vi "get 2d list.vi"(8 "error in (no error)":errorcluster, 10 "Y":u32[](array[numeric]), 11 "X":u32[](array[numeric])) -> (0 "error out (no error)":errorcluster, 1 "upper limit":dbl[](array[numeric]), 2 "lower limit":dbl[](array[numeric]), 4 "X Values":u32[](array[numeric]))   [LabVIEW 2016]
doc: "Takes X and Y create ROI values and confirms that all x values have two y values"
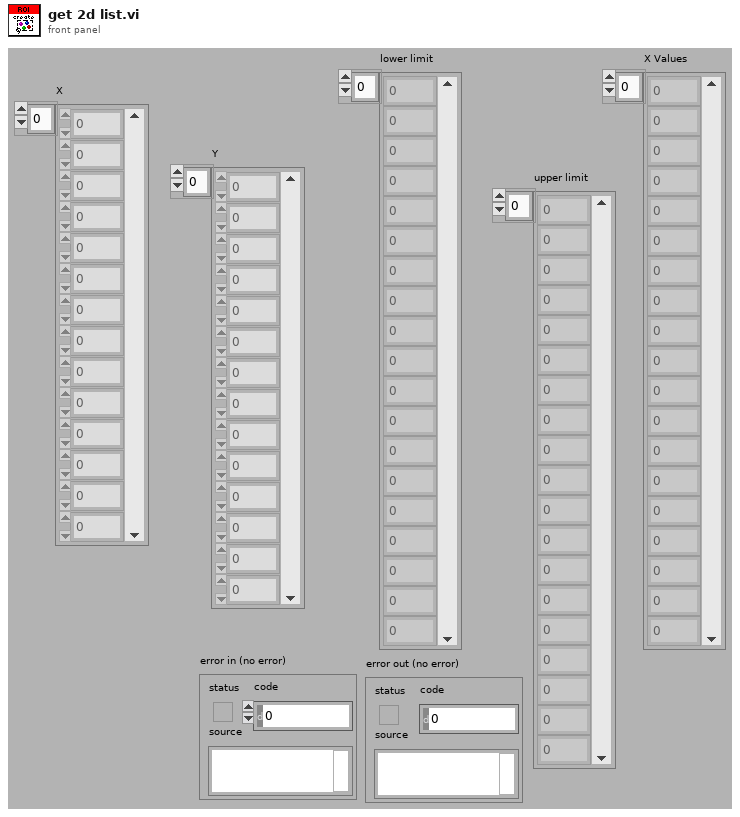
[diagram p1: front panel]
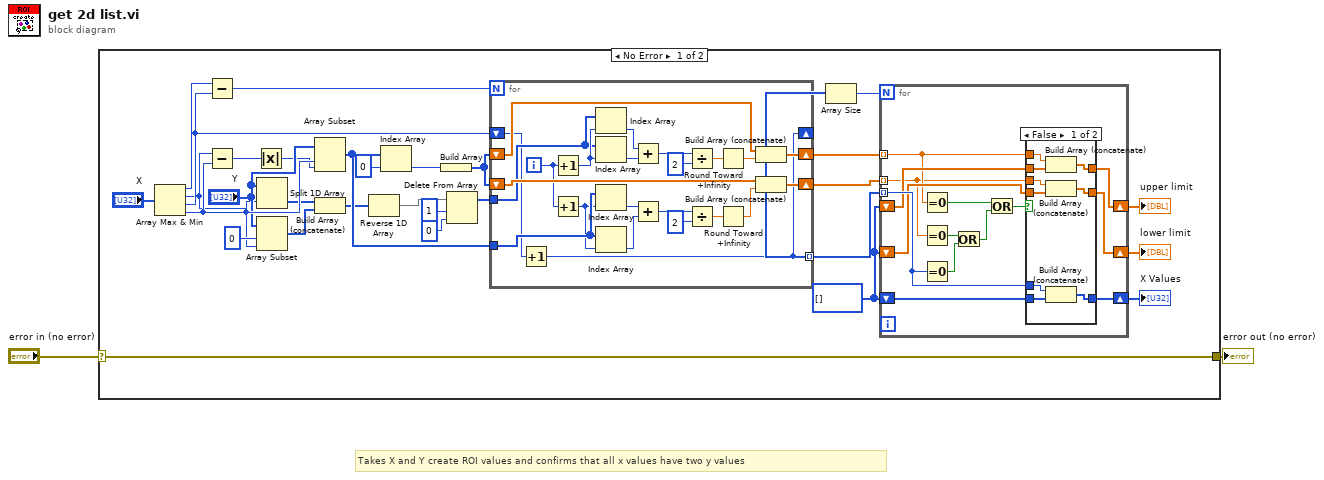
[diagram p0: block diagram]
diagram:
  # "Takes X and Y create ROI values and confirms that all x values have two y values"
  n1 = case shown="No Error" "error in (no error)" {
    selector: "error in (no error)" -> [w3 w82]
    tunnel: [w3 w82] -> w1
    frame No Error {
      w12 = u32[] []
      n2 = Array Max & Min(array="X") -> (max value=w14:u32, max index (indices)=w4:i32, min value=w15:u32, min index (indices)=w27:i32)
      n3 = Subtract(x=w14, y=w15) -> (x-y=w13:u32)
      n4 = Subtract(x=w4, y=w27) -> (x-y=w17:i32)
      n5 = Absolute Value(x=w17) -> (abs(x)=w16:i32)
      n6 = Split 1D Array(array="Y", index=w4) -> (second subarray=w23:u32[])  [unwired: 1 out]
      n7 = Array Subset(array="Y", index=0, length=w27) -> (w24:u32[])
      n8 = Array Subset(array="Y", index=w27, length=w16) -> (w31:u32[])
      n9 = Build Array (concatenate)(w23, w24) -> (w25:u32[])
      n10 = Reverse 1D Array(array=w25) -> (reversed array=w21:u32[])
      n11 = Index Array(array=w31, index=0) -> (element=w29:u32)
      n12 = Build Array(w29) -> (w22:u32[])
      n13 = Delete From Array(array=w21, length=1, index=0) -> (array with subset deleted=w18:u32[])  [unwired: 1 out]
      n14 = for {
        N: w13 -> [_]
        tunnel: w31 -> [w81]
        shift-right: [w75] -> w11
        shift-left: w22 -> [w72]
        shift-right: [w61] -> w10
        shift-left: w22 -> [w62]
        tunnel: w18 -> [w63]
        tunnel: [w59] -> w9 mode=indexing
        shift-right: [w59] -> _
        shift-left: w15 -> [w60]
        i -> [w65]
        n15 = Increment(x=w60) -> (x+1=w59:u32)
        n16 = Increment(x=w65) -> (x+1=w66:i32)
        n17 = Increment(x=w65) -> (x+1=w80:i32)
        n18 = Index Array(array=w63, index=w66) -> (element=w67:u32)
        n19 = Index Array(array=w63, index=w66) -> (element=w68:u32)
        n20 = Index Array(array=w81, index=w80) -> (element=w79:u32)
        n21 = Index Array(array=w81, index=w80) -> (element=w78:u32)
        n22 = Add(x=w67, y=w68) -> (x+y=w69:u32)
        n23 = Add(x=w79, y=w78) -> (x+y=w77:u32)
        n24 = Divide(x=w69, y=u32 2) -> (x/y=w71:dbl)
        n25 = Divide(x=w77, y=u32 2) -> (x/y=w74:dbl)
        n26 = Round Toward +Infinity(x=w71) -> (ceil(x): smallest int >= x=w64:dbl)
        n27 = Round Toward +Infinity(x=w74) -> (ceil(x): smallest int >= x=w73:dbl)
        n28 = Build Array (concatenate)(w62, w64) -> (w61:dbl[])
        n29 = Build Array (concatenate)(w72, w73) -> (w75:dbl[])
      }
      n30 = Array Size(array=w9) -> (size(s)=w8:i32)
      n31 = for {
        N: w8 -> [_]
        tunnel: w10 -> [w39] mode=indexing
        tunnel: w9 -> [w44] mode=indexing
        tunnel: w11 -> [w38] mode=indexing
        shift-right: [w46] -> w6
        shift-left: w12 -> [w42]
        shift-right: [w45] -> w7
        shift-left: w12 -> [w41]
        shift-right: [w43] -> w5
        shift-left: w12 -> [w40]
        n32 = Equal To 0?(x=w39) -> (x = 0?=w35:bool)
        n33 = Equal To 0?(x=w38) -> (x = 0?=w36:bool)
        n34 = Equal To 0?(x=w44) -> (x = 0?=w37:bool)
        n35 = Or(x=w36, y=w37) -> (x .or. y?=w34:bool)
        n36 = Or(x=w35, y=w34) -> (x .or. y?=w33:bool)
        n37 = case shown="False" w33 {
          tunnel: w39 -> [w55 _]
          tunnel: w38 -> [w52 _]
          tunnel: [w51 w57] -> w45
          tunnel: [w54 w58] -> w46
          tunnel: w44 -> [w49 _]
          tunnel: [w48 w56] -> w43
          tunnel: w42 -> [w53 w58]
          tunnel: w41 -> [w50 w57]
          tunnel: w40 -> [w47 w56]
          frame False {
            n38 = Build Array (concatenate)(w55, w53) -> (w54:dbl[])
            n39 = Build Array (concatenate)(w52, w50) -> (w51:dbl[])
            n40 = Build Array (concatenate)(w49, w47) -> (w48:u32[])
          }
          frame True {
          }
        }
      }
      "lower limit" <- w7
      "X Values" <- w5
      "upper limit" <- w6
    }
    frame Error {
    }
  }
  "error out (no error)" <- w1
